vi "RT_RAM.vi"() -> ()   [LabVIEW 2019]
uses:
  <vilib>/FPGAPlugInAG/myRIO-1900/niLvFpga_Open_myRIO-1900.vi
  <vilib>/rvi/interface/common/dynamic/niFpgaDynamicAddResources.vi
  <vilib>/Utility/error.llb/Error Cluster From Error Code.vi
  <vilib>/rvi/errors/niLvFpgaAdjustHostInterfaceError.vi
  <vilib>/FPGAPlugInAG/Dynamic/niLvFpga_Run_Dynamic.vi
  <vilib>/FPGAPlugInAG/Dynamic/niLvFpga_Close_Dynamic.vi
  <vilib>/rvi/interface/nirviOpenFPGA/nirviOpenFPGA.xnode
  FPGA Bitfiles/karolinasawosz_FPGATarget_AccXnew_J55o-5fcSn8.lvbitx
  AccX_new.vi
  <vilib>/rvi/interface/nirviMethod/nirviMethod.xnode
  <vilib>/rvi/interface/nirviReadWriteControl/nirviReadWriteControl.xnode
  <vilib>/rvi/interface/nirviCloseFPGA/nirviCloseFPGA.xnode
  <vilib>/rvi/errors/niLvFpgaMergeErrorWithErrorCode.vi
  <vilib>/FPGAPlugInAG/Dynamic/niLvFpga_ReadFifo_Dynamic.vi
  <vilib>/FPGAPlugInAG/Dynamic/niLvFpga_StartFifo_Dynamic.vi
  NiFpgaLv.dll
  <vilib>/rvi/interface/Simulation/niFpgaSimulationCallBeginRW.vi
panel:
  out "Elements Remaining":u32
  out "error out":errorcluster
  out "Waveform Graph":i16[][](graph)
  in  "stop":bool
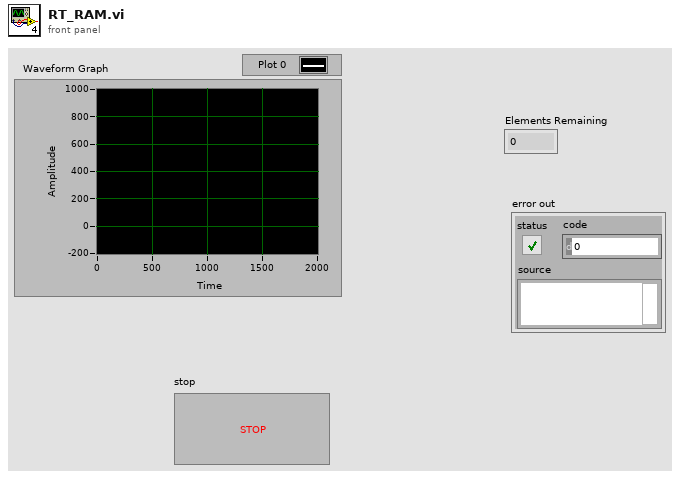
[diagram p1: front panel]
types:
  T1 = cluster{"XDiscrimination":i16, "YDiscrimination":i16, "ZDiscrimination":i16}
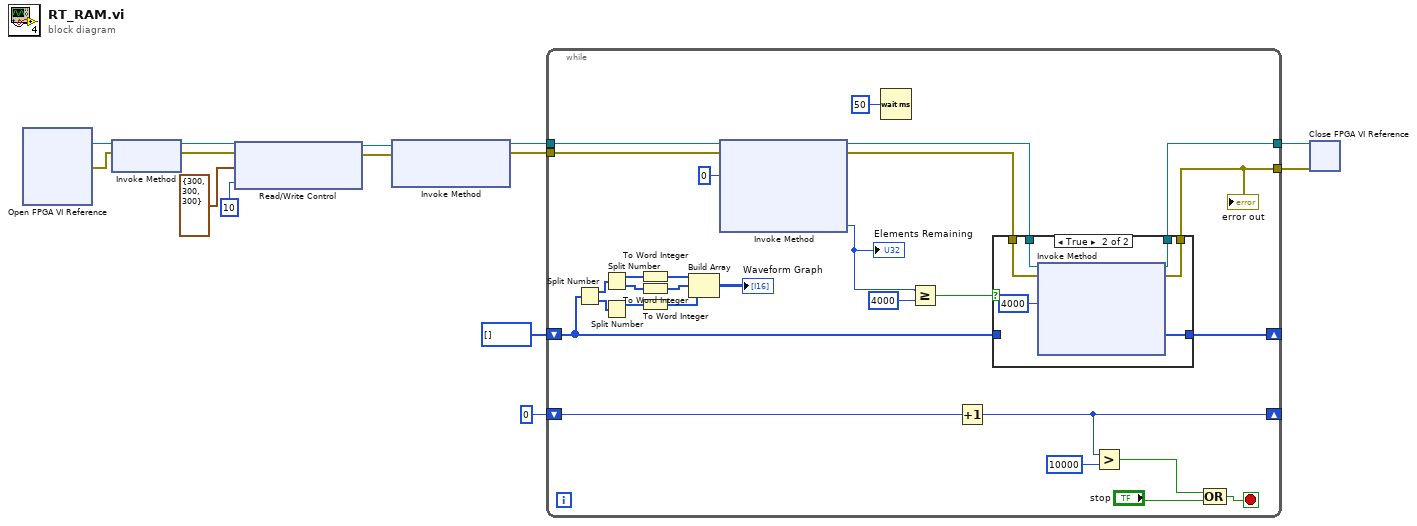
[diagram p0: block diagram]
diagram:
  n1 = xnode "Open FPGA VI Reference"() -> ("FPGA VI Reference Out"=w12:refnum<k20>, "error out"=w11:errorcluster)  [unwired: 2 in]
  n2 = xnode "Invoke Method"("FPGA VI Reference In"=w12, "error in"=w11) -> ("FPGA VI Reference Out"=w4:refnum<k20>, "error out"=w3:errorcluster)
  n3 = xnode "Read/Write Control"("FPGA VI Reference In"=w4, "error in"=w3, "Discrimination levels"=T1 {"XDiscrimination"=300, "YDiscrimination"=300, "ZDiscrimination"=300}, "Samples amount"=i16 10) -> ("FPGA VI Reference Out"=w2:refnum<k20>, "error out"=w1:errorcluster)
  n4 = xnode "Invoke Method"("FPGA VI Reference In"=w2, "error in"=w1) -> ("FPGA VI Reference Out"=w10:refnum<k20>, "error out"=w9:errorcluster)  [unwired: 1 in]
  n5 = while {
    shift-right: [w40] -> _
    shift-left: i16 0 -> [w36]
    tunnel: [w31] -> w13
    tunnel: w10 -> [w16]
    tunnel: w9 -> [w15]
    tunnel: [w29] -> w8
    shift-right: [w18] -> _
    shift-left: u64[] [] ("Data") -> [w17]
    stop <- w37 stop-if-true
    n6 = Split Number(x=w17) -> (hi(x)=w27:u32[], lo(x)=w26:u32[])
    n7 = Split Number(x=w27) -> (hi(x)=w23:u16[], lo(x)=w24:u16[])
    n8 = Split Number(x=w26) -> (hi(x)=w25:u16[])  [unwired: 1 out]
    n9 = To Word Integer(number=w23) -> (16bit integer=w21:i16[])
    n10 = To Word Integer(number=w24) -> (16bit integer=w20:i16[])
    n11 = To Word Integer(number=w25) -> (16bit integer=w19:i16[])
    n12 = Build Array(w21, w20, w19) -> (→"Waveform Graph":i16[][])
    n13 = xnode "Invoke Method"("FPGA VI Reference In"=w16, "error in"=w15, "Number of Elements"=u32 0) -> ("FPGA VI Reference Out"=w32:refnum<k20>, "error out"=w30:errorcluster, "Elements Remaining"=w35:u32)  [unwired: 1 in, 1 out]
    "Elements Remaining" <- w35
    n14 = Wait (ms)(milliseconds to wait=u32 50) -> ()  [unwired: 1 out]
    n15 = Greater Or Equal?(x=w35, y=u32 4000) -> (x >= y?=w33:bool)
    n16 = Increment(x=w36) -> (x+1=w40:i16)
    n17 = case shown="True" w33 {
      tunnel: w32 -> [w45 w51]
      tunnel: [w45 w50] -> w31
      tunnel: w30 -> [w44 w49]
      tunnel: [w44 w48] -> w29
      tunnel: [w43 w46] -> w18
      tunnel: w17 -> [w43 _]
      frame False {
      }
      frame True {
        n18 = xnode "Invoke Method"("FPGA VI Reference In"=w51, "error in"=w49, "Number of Elements"=u32 4000) -> ("FPGA VI Reference Out"=w50:refnum<k20>, "error out"=w48:errorcluster, "Data"=w46:u64[])  [unwired: 1 in, 1 out]
      }
    }
    "error out" <- w29
    n19 = Greater?(x=w40, y=i16 10000) -> (0:w38:bool)
    n20 = Compound Arithmetic op=OR(w38, "stop") -> (w37:bool)
  }
  n21 = xnode "Close FPGA VI Reference"("FPGA VI Reference In"=w13, "error in"=w8) -> ()  [unwired: 1 out]
